vi "MFC_StringFormat.vi"(11 "Array":string[](array[string])) -> (3 "Array out":T1(array[cluster]) {"Setpoint" format="%.2f"; "MassFlow" format="%.2f"})   [LabVIEW 2014]
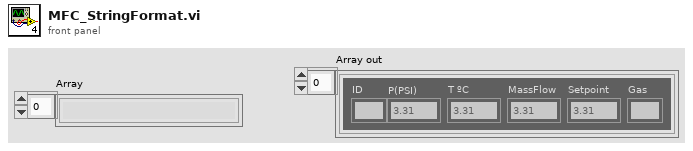
[diagram p1: front panel]
types:
  T1 = cluster{"ID":string, "P(PSI)":dbl, "T ºC":dbl, "MassFlow":dbl, "Setpoint":dbl, "Gas":string}[]
  T2 = cluster{"ID":string, "P(PSI)":dbl, "T ºC":dbl, "MassFlow":dbl, "Setpoint":dbl, "Gas":string}
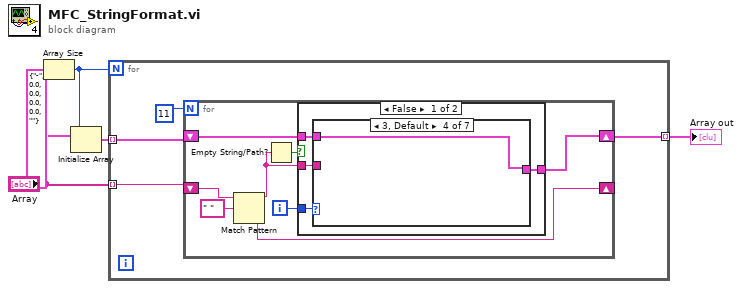
[diagram p0: block diagram]
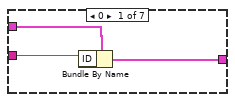
[diagram p2: hidden frame]
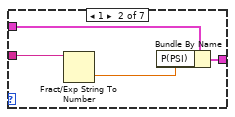
[diagram p3: hidden frame]
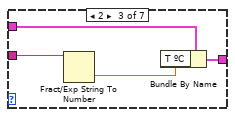
[diagram p4: hidden frame]
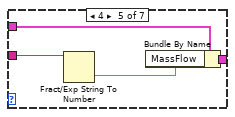
[diagram p5: hidden frame]
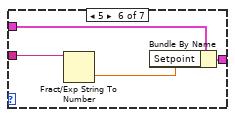
[diagram p6: hidden frame]
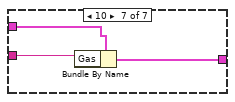
[diagram p7: hidden frame]
diagram:
  n1 = Array Size(array="Array") -> (size(s)=w2:i32)
  n2 = Initialize Array(T2 {"ID"="-", "P(PSI)"=0.0, "T ºC"=0.0, "MassFlow"=0.0, "Setpoint"=0.0, "Gas"=""} ("MFC data"), w2) -> (w1:T1)
  n3 = for {
    N: w2 -> [_]
    tunnel: [w8] -> w5 mode=indexing
    tunnel: "Array" -> [w7] mode=indexing
    tunnel: w1 -> [w6] mode=indexing
    n4 = for {
      N: 11 ("Numeric") -> [_]
      shift-right: [w15] -> _
      shift-left: w7 -> [w17]
      shift-right: [w10] -> w8
      shift-left: w6 -> [w12]
      i -> [w11]
      n5 = Match Pattern(string=w17, regular expression=" ") -> (before substring=w13:string, after substring=w15:string)  [unwired: 1 in, 2 out]
      n6 = Empty String/Path?(string/path=w13) -> (empty?=w14:bool)
      n7 = case shown="False" w14 {
        tunnel: w13 -> [w18 _]
        tunnel: w12 -> [w21 w45]
        tunnel: w11 -> [w20 _]
        tunnel: [w19 w45] -> w10
        frame False {
          n8 = case shown="3, Default" w20 {
            tunnel: w21 -> [w24 w28 w32 w33 w37 w41 w44]
            tunnel: [w23 w27 w31 w33 w36 w40 w43] -> w19
            tunnel: w18 -> [w22 w26 w30 _ w35 w39 w42]
            frame 0 {
              n9 = Bundle By Name(cluster=w24, "ID"=w22) -> (w23:T2)
            }
            frame 1 {
              n10 = Fract/Exp String To Number(string=w26) -> (number=w25:dbl)  [unwired: 3 in, 1 out]
              n11 = Bundle By Name(cluster=w28, "P(PSI)"=w25) -> (w27:T2)
            }
            frame 2 {
              n12 = Fract/Exp String To Number(string=w30) -> (number=w29:dbl)  [unwired: 3 in, 1 out]
              n13 = Bundle By Name(cluster=w32, "T ºC"=w29) -> (w31:T2)
            }
            frame 3, Default {
            }
            frame 4 {
              n14 = Fract/Exp String To Number(string=w35) -> (number=w34:dbl)  [unwired: 3 in, 1 out]
              n15 = Bundle By Name(cluster=w37, "MassFlow"=w34) -> (w36:T2)
            }
            frame 5 {
              n16 = Fract/Exp String To Number(string=w39) -> (number=w38:dbl)  [unwired: 3 in, 1 out]
              n17 = Bundle By Name(cluster=w41, "Setpoint"=w38) -> (w40:T2)
            }
            frame 10 {
              n18 = Bundle By Name(cluster=w44, "Gas"=w42) -> (w43:T2)
            }
          }
        }
        frame True {
        }
      }
    }
  }
  "Array out" <- w5
